vi "acquireValue.vi"(8 "error in (no error)":errorcluster, 10 "nextSample?":bool, 11 "mainDoorState in":refnum<class "mainDoorState.lvclass">) -> (0 "error out":errorcluster, 1 "function return":i32, 2 "variantData":variant, 3 "mainDoorState out":refnum<class "mainDoorState.lvclass">)   [LabVIEW 2016, in "SALLV_AtDome_Messaging.lvlib" / "mainDoorState.lvclass"]
uses:
  mainDoorState.lvclass
  ts_sallv_AtDome/SALLV_AtDome.lvlib
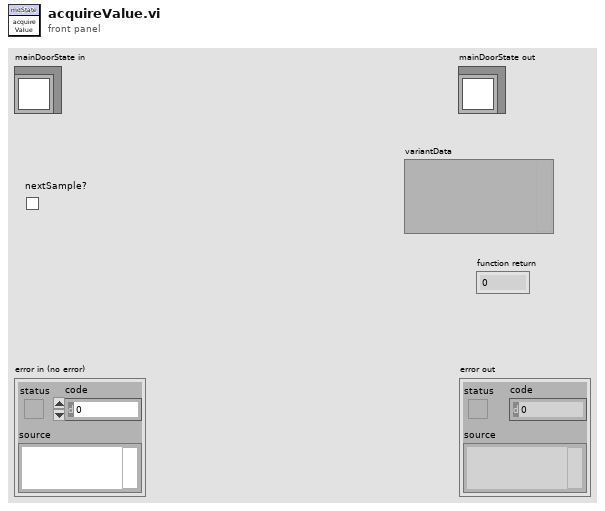
[diagram p1: front panel]
types:
  T1 = typedef "SALLV_AtDome.lvlib/logevent_mainDoorState.ctl" = cluster{"state":i32, "priority":i32}
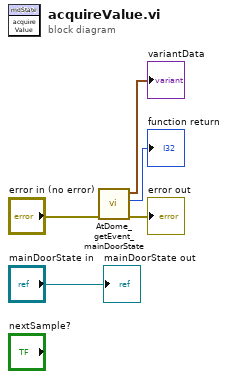
[diagram p0: block diagram]
diagram:
  n1 = call "AtDome_getEvent_mainDoorState.vi"("error in (no error)"="error in (no error)") -> ("error out"=→"error out":errorcluster, "function return"=→"function return":i32, "logevent_mainDoorState_Ctl out"=→"variantData":T1)  [unwired: 8 in]
  "mainDoorState out" <- "mainDoorState in"
